vi "Counts_LSW_edits.vi"() -> ()   [LabVIEW 2015]
doc: "This sample project is built upon the standard state machine template and shows how you could create an application that acquires, analyzes, and presents data. It includes functionality for presenting configuration dialogs, preserving settings between executions, loading and saving data, as well as exporting graph images and text files.\n\nIt is most appropriate for data that is acquired instantly as it does not allow for screen updates mid acquisition nor does it allow for continuous streaming to disk."
uses:
  <vilib>/ptbypt/NI_PtbyPt.lvlib
panel:
  out "freq multiplier...":dbl
  out "Seconds":dbl
  out "Counts":dbl
  in  "Runs":dbl=100.0
  in  "Pulse TTL 2":bool
  in  "Pulse TTL 1":bool
  in  "Toggle\nTTL 2":bool
  in  "Toggle\nTTL 1":bool
  in  "Record\nstatistics":bool
  in  "Raw Data\nFile Name 2":string="C:\\FPGA\\stats.txt"
  in  "Clock Freq. [MHz]":dbl=48.0
  in  "Record\nraw data":bool
  out "Elapsed time (s)":dbl
  out "FPGA Counts\nStatus":dbl
  out "USB Open\nStatus":dbl
  out "Channel 4 Total\nCounts":dbl
  out "Channel 3 Total\nCounts":dbl
  out "Channel 2 Total\nCounts":dbl
  out "Channel 1 Total\nCounts":dbl
  in  "Raw Data\nFile Name":string="C:\\FPGA\\raw.txt"
  out "?":dbl
  out "?":dbl
  out "?":dbl
  out "?":dbl
  out "stats":i64[](array[numeric])
  in  "Stop":bool
  out "Channel 4 CPS":dbl(knob) scale=0.0..1000000.0
  out "Channel 3 CPS":dbl(knob) scale=0.0..1000000.0
  out "Channel 2 CPS":dbl(knob) scale=0.0..1000000.0
  out "Channel 1 CPS":dbl(knob) scale=0.0..1000000.0
  # "Clocks"
  # "Channel 1"
  # "Channel 2"
  # "Channel 3"
  # "Channel 4"
  # "Coincidence Channels 1 & 2"
  # "Coincidence Channels 1 & 3"
  # "Coincidence Channels 1 & 4"
  # "Coincidence Channels 2 & 3"
  # "Coincidence Channels 2 & 4"
  # "Coincidence Channels 3 & 4"
  # "Coincidence Channels 1 & 2 & 3"
  # "Coincidence Channels 1 & 2 & 4"
  # "Coincidence Channels 1 & 3 & 4"
  # "Coincidence Channels 2 & 3 & 4"
  # "Coincidence Channels 1 & 2 & 3 & 4"
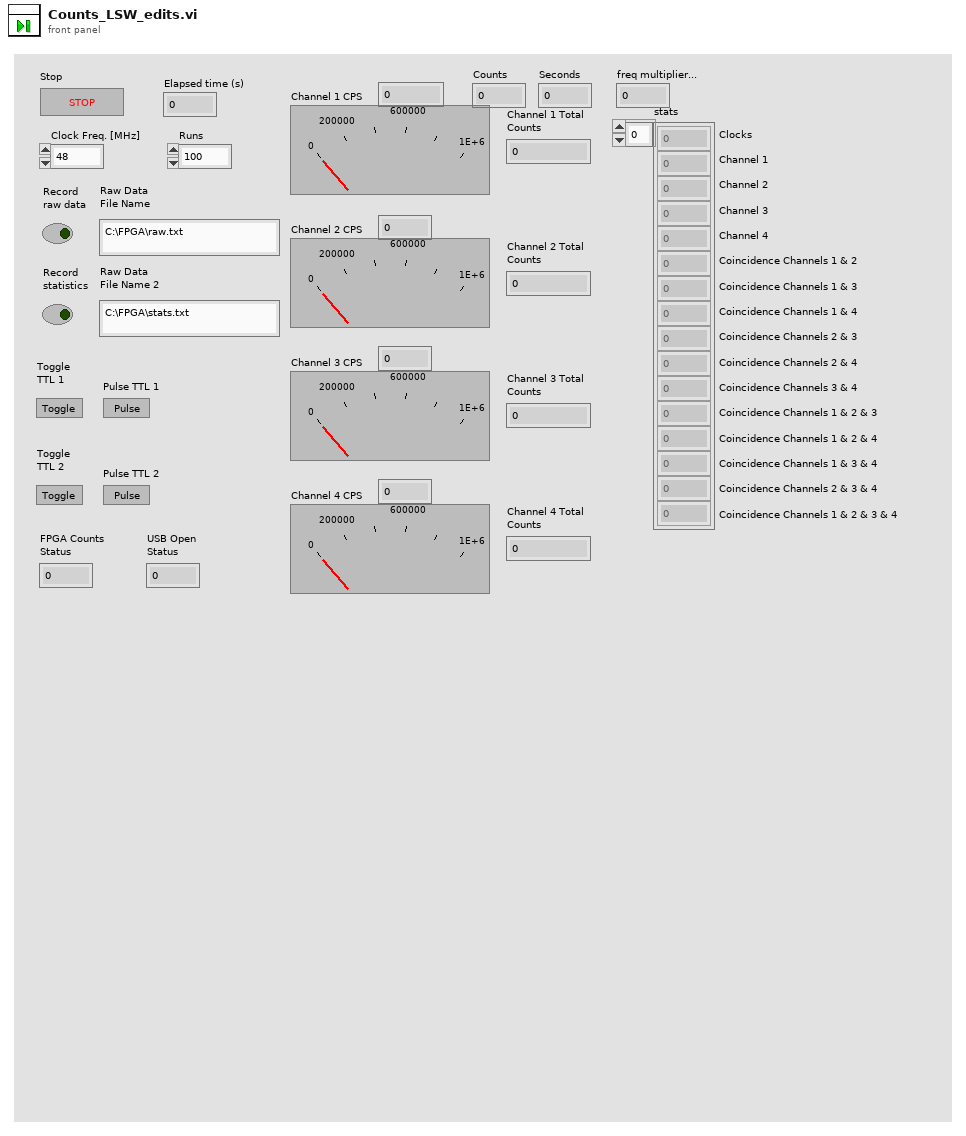
[diagram p1: front panel]
types:
  T1 = enum16{"open", "replace", "create", "open or create", "replace or create", "replace or create with confirmation"}
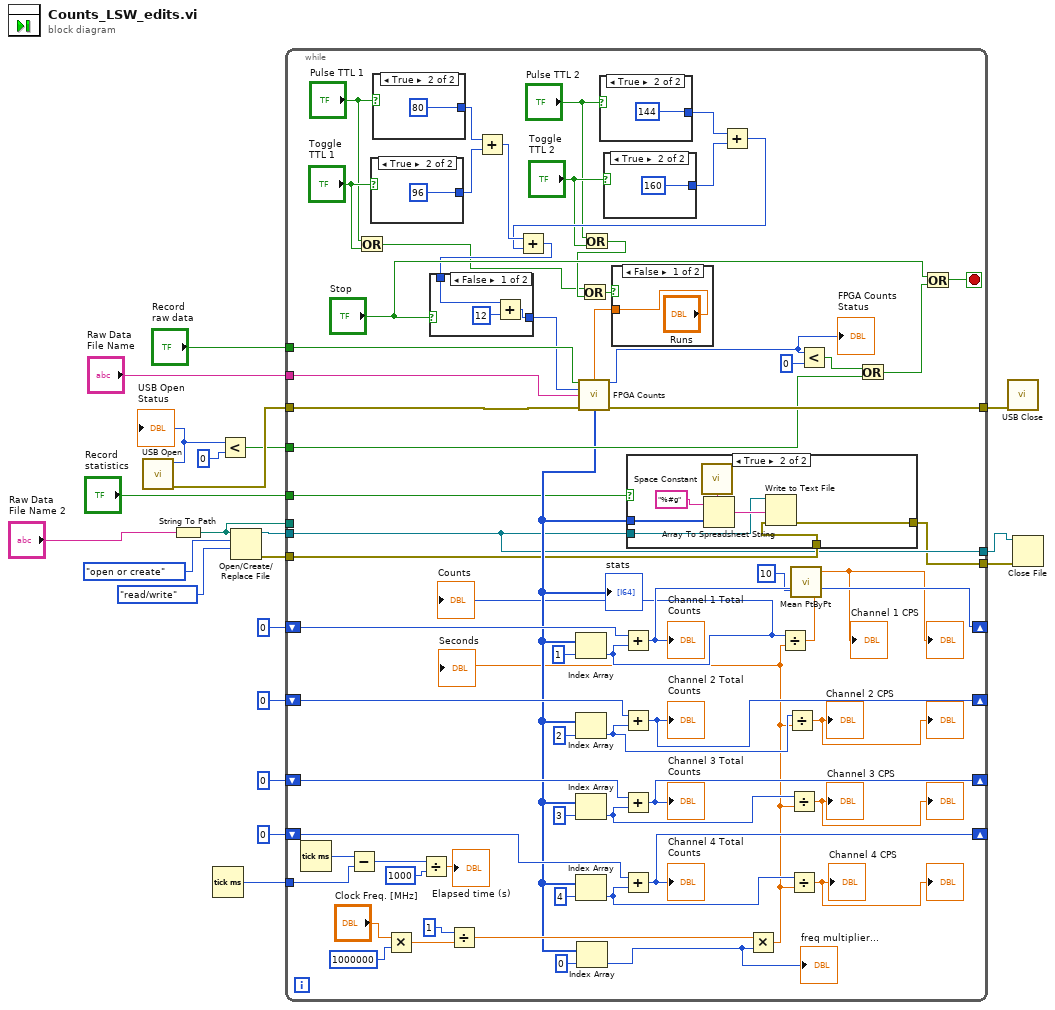
[diagram p0: block diagram]
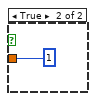
[diagram p2: hidden frame]
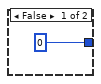
[diagram p3: hidden frame]
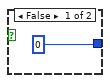
[diagram p4: hidden frame]
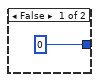
[diagram p5: hidden frame]
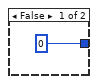
[diagram p6: hidden frame]
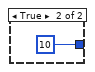
[diagram p8: hidden frame]
diagram:
  n1 = call "USB Open.vi"() -> ("error out"=w15:errorcluster, "function return"=w12:i32)  [unwired: 10 in]
  "USB Open\nStatus" <- w12
  n2 = String To Path(string="Raw Data\nFile Name 2") -> (path=w4:path)
  n3 = Tick Count (ms)() -> (millisecond timer value=w10:u32)
  n4 = Less?(x=w12, y=0) -> (x < y?=w11:bool)
  n5 = Open/Create/Replace File(file path (use dialog)=w4, operation (0:open)=T1."open or create", access (0:read/write)=enum16{"read/write", "read-only", "write-only"}."read/write") -> (refnum out=w3:refnum<file>, error out=w5:errorcluster)  [unwired: 3 in, 1 out]
  n6 = while {
    shift-right: [w28] -> _
    shift-left: 0 -> [w79]
    shift-right: [w53] -> _
    shift-left: 0 -> [w80]
    shift-right: [w52] -> _
    shift-left: 0 -> [w81]
    shift-right: [w51] -> _
    shift-left: 0 -> [w82]
    tunnel: w15 -> [w29]
    tunnel: [w61] -> w14
    tunnel: "Record\nraw data" -> [w63]
    tunnel: "Raw Data\nFile Name" -> [w60]
    tunnel: w11 -> [w57]
    tunnel: w10 -> [w50]
    tunnel: "Record\nstatistics" -> [w47]
    tunnel: w5 -> [w46]
    tunnel: w4 -> [_]
    tunnel: w3 -> [w45]
    tunnel: [w45] -> w2
    tunnel: [w44] -> w1
    stop <- w54 stop-if-true
    n7 = Tick Count (ms)() -> (millisecond timer value=w70:u32)
    n8 = Subtract(x=w70, y=w50) -> (x-y=w88:u32)
    n9 = Or(x="Pulse TTL 1", y="Toggle\nTTL 1") -> (x .or. y?=w30:bool)
    n10 = case shown="True" "Toggle\nTTL 1" {
      tunnel: [0 96] -> w42
      frame False {
      }
      frame True {
      }
    }
    n11 = case shown="True" "Pulse TTL 1" {
      tunnel: [0 80] -> w43
      frame False {
      }
      frame True {
      }
    }
    n12 = Multiply(x="Clock Freq. [MHz]", y=1000000) -> (x*y=w69:dbl)
    n13 = Divide(x=w88, y=1000) -> (x/y=→"Elapsed time (s)":dbl)
    n14 = Divide(x=1, y=w69) -> (x/y=w67:dbl)
    n15 = Add(x=w43, y=w42) -> (x+y=w41:i32)
    n16 = Or(x="Pulse TTL 2", y="Toggle\nTTL 2") -> (x .or. y?=w35:bool)
    n17 = Or(x=w30, y=w35) -> (x .or. y?=w36:bool)
    n18 = case shown="True" "Pulse TTL 2" {
      tunnel: [0 144] -> w38
      frame False {
      }
      frame True {
      }
    }
    n19 = case shown="True" "Toggle\nTTL 2" {
      tunnel: [0 160] -> w39
      frame False {
      }
      frame True {
      }
    }
    n20 = case shown="False" w36 {
      tunnel: ["Runs" 1] -> w62
      frame False {
      }
      frame True {
      }
    }
    n21 = Add(x=w38, y=w39) -> (x+y=w37:i32)
    n22 = Add(x=w41, y=w37) -> (x+y=w40:i32)
    n23 = case shown="False" "Stop" {
      tunnel: [w108 10] -> w58
      tunnel: w40 -> [w107 _]
      frame False {
        n24 = Add(x=w107, y=12) -> (x+y=w108:i32)
      }
      frame True {
      }
    }
    n25 = call "FPGA Counts.vi"("saveData"=w63, "runs"=w62, "fpgaCommand"=w58, "fileName"=w60, "error in (no error)"=w29) -> ("function return"=w59:i32, "stats"=w48:i64[], "error out"=w61:errorcluster)  [unwired: 6 in, 2 out]
    "stats" <- w48
    "FPGA Counts\nStatus" <- w59
    n26 = Index Array(array=w48, index=1) -> (element=w27:i64)
    "Counts" <- w27
    n27 = Index Array(array=w48, index=2) -> (element=w73:i64)
    n28 = Index Array(array=w48, index=3) -> (element=w72:i64)
    n29 = Index Array(array=w48, index=4) -> (element=w71:i64)
    n30 = Index Array(array=w48, index=0) -> (element=w25:i64)
    "freq multiplier..." <- w25
    n31 = Add(x=w79, y=w27) -> (x+y=w28:i64)
    "Channel 1 Total\nCounts" <- w28
    n32 = Add(x=w80, y=w73) -> (x+y=w53:i64)
    "Channel 2 Total\nCounts" <- w53
    n33 = Add(x=w81, y=w72) -> (x+y=w52:i64)
    "Channel 3 Total\nCounts" <- w52
    n34 = Add(x=w82, y=w71) -> (x+y=w51:i64)
    "Channel 4 Total\nCounts" <- w51
    n35 = case shown="True" w47 {
      tunnel: w48 -> [_ w104]
      tunnel: w46 -> [w99 w101]
      tunnel: w45 -> [_ w102]
      tunnel: [w99 w100] -> w44
      frame False {
      }
      frame True {
        n36 = call <vilib>:"Space Constant.vi"() -> ("String"=w106:string)
        n37 = Array To Spreadsheet String(delimiter (Tab)=w106, array=w104, 3:"%#g") -> (spreadsheet string=w103:string)
        n38 = Write to Text File(file (use dialog)=w102, text=w103, error in=w101) -> (error out=w100:errorcluster)  [unwired: 1 in, 2 out]
      }
    }
    n39 = Multiply(x=w67, y=w25) -> (x*y=w26:dbl)
    "Seconds" <- w26
    n40 = Divide(x=w27, y=w26) -> (x/y=w24:dbl)
    n41 = Divide(x=w73, y=w26) -> (x/y=→"Channel 2 CPS" →"?":dbl)
    n42 = Divide(x=w72, y=w26) -> (x/y=→"Channel 3 CPS" →"?":dbl)
    n43 = Divide(x=w71, y=w26) -> (x/y=→"Channel 4 CPS" →"?":dbl)
    n44 = call <vilib>:"Mean PtByPt.vi"("x"=w24, "sample length"=10) -> ("mean"=→"Channel 1 CPS" →"?":dbl)  [unwired: 2 in, 1 out]
    n45 = Less?(x=w59, y=0) -> (x < y?=w56:bool)
    n46 = Or(x=w56, y=w57) -> (x .or. y?=w55:bool)
    n47 = Or(x="Stop", y=w55) -> (x .or. y?=w54:bool)
  }
  n48 = call "USB Close.vi"("error in (no error)"=w14) -> ()  [unwired: 9 in, 2 out]
  n49 = Close File(refnum=w2, error in=w1) -> ()  [unwired: 2 out]
